vi "NI VeriStand - Report Error.vi"(8 "error in (no error)":errorcluster, 9 "New Error":errorcluster, 10 "Error ID":string, 11 "Node Ref in":T1 format="%.0x") -> (0 "error out":errorcluster, 3 "Node Ref out":T1=18446744073709551615 format="%.0x")   [LabVIEW 2020, in "Custom Device Offline API.lvlib"]
uses:
  <vilib>/NI VeriStand/Custom Device Offline API/Custom Device Offline API.lvlib
  <vilib>/NI VeriStand/Custom Device API/Custom Device Item Ref.ctl
  NationalInstruments.VeriStand.SystemDefinitionAPI
  <vilib>/NI VeriStand/Custom Device API/Custom Device API.lvlib
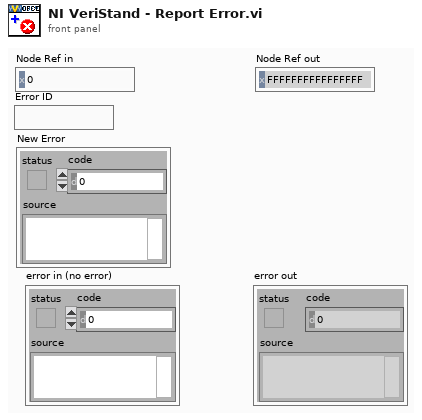
[diagram p1: front panel]
types:
  T1 = typedef "Custom Device API.lvlib/Custom Device Item Ref.ctl" = u64
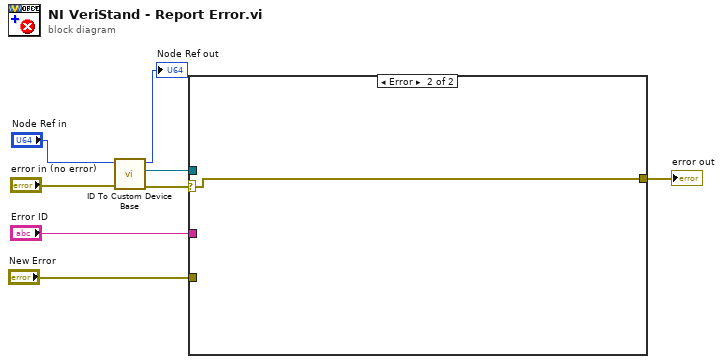
[diagram p0: block diagram]
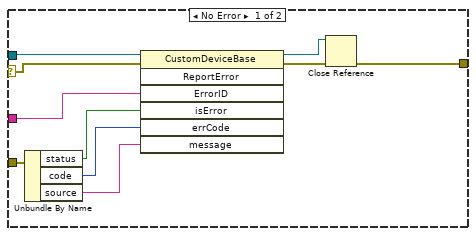
[diagram p2: hidden frame]
diagram:
  n1 = call <vilib>:"ID To Custom Device Base.vi"("error in (no error)"="error in (no error)", "ID in"="Node Ref in") -> ("error out"=w6:errorcluster, "BaseNode"=w5:refnum<k24>, "ID out"=→"Node Ref out":u64)  [unwired: 7 in]
  n2 = case shown="Error" w6 {
    selector: w6 -> [w16 w19]
    tunnel: w5 -> [w18 _]
    tunnel: "Error ID" -> [w17 _]
    tunnel: "New Error" -> [w15 _]
    tunnel: [w9 w19] -> w1
    frame No Error {
      n3 = Unbundle By Name(w15) -> ("status"=w14:bool, "code"=w13:i32, "source"=w12:string)
      n4 = invoke class="CustomDeviceBase" method="ReportError"(reference=w18, error in=w16, "ErrorID"=w17, "isError"=w14, "errCode"=w13, "message"=w12) -> (reference out=w10:refnum<k24>, error out=w11:errorcluster)  [unwired: 1 in, 5 out]
      n5 = Close Reference(reference=w10, error in (no error)=w11) -> (error out=w9:errorcluster)
    }
    frame Error {
    }
  }
  "error out" <- w1
